vi "pl1000OpenUnit.vi"(8 "error in (no error)":errorcluster) -> (0 "error out":errorcluster, 3 "pl1000 handle out":i16)   [LabVIEW 2010]
uses:
  pl1000.dll
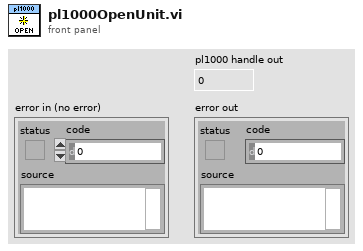
[diagram p1: front panel]
types:
  T1 = cluster{"status":bool, "code":u32, "source":string}
  T2 = cluster{"status":bool, "code":bool, "source":bool}
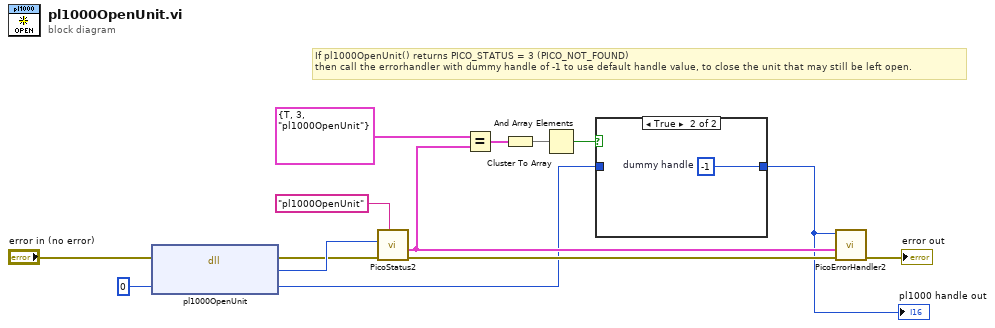
[diagram p0: block diagram]
diagram:
  # "If pl1000OpenUnit() returns PICO_STATUS = 3 (PICO_NOT_FOUND)\nthen call the errorhandler with dummy handle of -1 to use default handle value, to close the unit that may still be left open."
  n1 = dll-call lib="pl1000.dll" fn="pl1000OpenUnit"(error in="error in (no error)", "handle"=i16 0) -> (error out=w11:errorcluster, "status"=w12:u32, "handle"=w3:i16)  [unwired: 2 in, 1 out]
  n2 = call "PicoStatus2.vi"("PICO source"="pl1000OpenUnit", "Error in"=w11, "PICO STATUS"=w12) -> ("error out"=w6:errorcluster, "PICO_STATUS out"=w5:T1)  [unwired: 5 in]
  n3 = Equal?(x=T1 {"status"=TRUE, "code"=3, "source"="pl1000OpenUnit"} ("PICO_STATUS out"), y=w5) -> (x = y?=w9:T2)
  n4 = Cluster To Array(cluster=w9) -> (array=w8:bool[])
  n5 = And Array Elements(Boolean array=w8) -> (logical AND=w4:bool)
  n6 = case shown="True" w4 {
    tunnel: w3 -> [w15 _]
    tunnel: [w15 w16] -> w2
    frame False {
    }
    frame True {
      w16 = i16 -1  # dummy handle
    }
  }
  "pl1000 handle out" <- w2
  n7 = call "PicoErrorHandler2.vi"("error in (no error)"=w6, "PICO_STATUS in"=w5, "handle In"=w2) -> ("error out"=→"error out":errorcluster)  [unwired: 8 in]
